vi "obtainSALLVFunctionReferences.vi"(8 "error in (no error)":errorcluster, 11 "rejectedCommand in":refnum<class "rejectedCommand.lvclass">) -> (0 "error out":errorcluster, 3 "rejectedCommand out":refnum<class "rejectedCommand.lvclass">)   [LabVIEW 2016, in "SALLV_MtAtElectrometer_Messaging.lvlib" / "rejectedCommand.lvclass"]
uses:
  rejectedCommand.lvclass
  home/andres/ts_electrometer2/SALTopic/SALTopic/SALTopic.lvclass
  rejectedCommand.lvclass/rejectedCommand.ctl
  SALTopic/SALEvent/SALEvent.lvclass
  SALTopic/SALTopic/SALTopic.lvclass
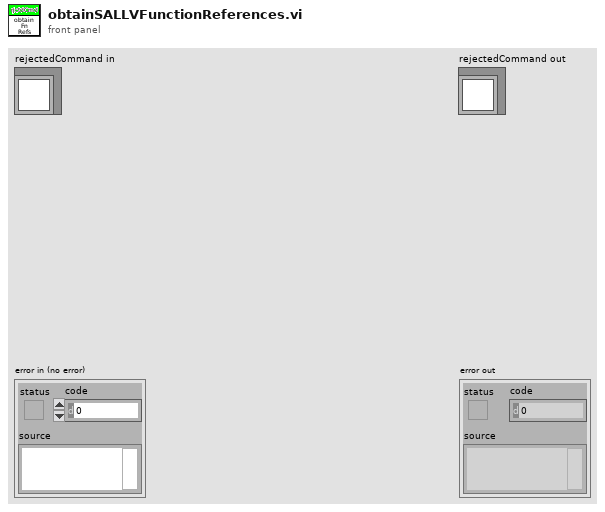
[diagram p1: front panel]
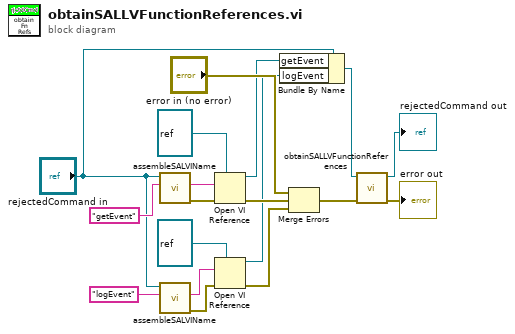
[diagram p0: block diagram]
diagram:
  n1 = call "assembleSALVIName.vi"("topicKey"="getEvent" ("commandKey"), "SALTopic in"="rejectedCommand in") -> ("error out"=w14:errorcluster, "viPath"=w15:string)  [unwired: 7 in, 1 out]
  n2 = call "assembleSALVIName.vi"("topicKey"="logEvent" ("commandKey"), "SALTopic in"="rejectedCommand in") -> ("error out"=w11:errorcluster, "viPath"=w10:string)  [unwired: 7 in, 1 out]
  n3 = Open VI Reference(type specifier VI Refnum (for type only)=refnum<vi> refnum ("reference"), vi path=w15, error in (no error)=w14) -> (vi reference=w2:refnum<vi>, error out=w5:errorcluster)  [unwired: 3 in]
  n4 = Open VI Reference(type specifier VI Refnum (for type only)=refnum<vi> refnum ("reference"), vi path=w10, error in (no error)=w11) -> (vi reference=w1:refnum<vi>, error out=w4:errorcluster)  [unwired: 3 in]
  n5 = Bundle By Name(cluster="rejectedCommand in", "getEvent"=w2, "logEvent"=w1) -> (w7:refnum<class "rejectedCommand.lvclass">)
  n6 = Merge Errors("error in (no error)", w5, w4) -> (w3:errorcluster)
  n7 = call-parent "obtainSALLVFunctionReferences.vi"("error in (no error)"=w3, "SALEvent in"=w7) -> ("error out"=→"error out":errorcluster, "SALEvent out"=→"rejectedCommand out":refnum<class "rejectedCommand.lvclass">)  [unwired: 8 in]
